vi "Wrap.vi"(7 "increment amount (1)":i32=1, 10 "mask":i32, 11 "index":i32) -> (3 "wrapped":i32)   [LabVIEW 2024, in "POTTypedCircularBuffer.lvclass"]
uses:
  POTTypedCircularBuffer.lvclass
  POTTypedCircularBuffer.lvclass/POTTypedCircularBuffer.ctl
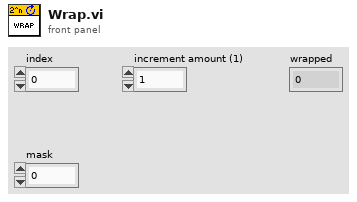
[diagram p1: front panel]
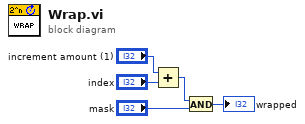
[diagram p0: block diagram]
diagram:
  n1 = Add(x="increment amount (1)", y="index") -> (x+y=w2:i32)
  n2 = And(x=w2, y="mask") -> (x .and. y?=→"wrapped":i32)
